vi "Module ID.vi"(11 "Module in":refnum<class "Module.lvclass">) -> (2 "Module ID":string)   [LabVIEW 2020, in "Volatus.lvlib" / "Module.lvclass"]
uses:
  Module.lvclass
  Module.lvclass/Module.ctl
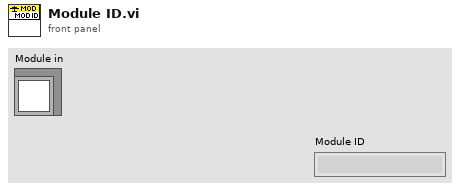
[diagram p1: front panel]
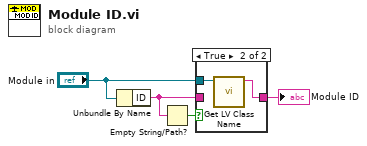
[diagram p0: block diagram]
diagram:
  n1 = Unbundle By Name("Module in") -> ("ID"=w3:string)
  n2 = Empty String/Path?(string/path=w3) -> (empty?=w4:bool)
  n3 = case shown="True" w4 {
    tunnel: w3 -> [w5 _]
    tunnel: "Module in" -> [_ w7]
    tunnel: [w5 w6] -> w2
    frame False {
    }
    frame True {
      n4 = call <vilib>:"Get LV Class Name.vi"("object"=w7) -> ("class name"=w6:string)  [unwired: 9 in, 1 out]
    }
  }
  "Module ID" <- w2
